vi "Linear Fit correlation.vi"(0 "Y Values":dbl[](array[numeric]) format="%.2f", 1 "X Values":dbl[](array[numeric]) format="%.2f") -> (2 "slope":dbl format="%.2f", 3 "intercept":dbl format="%.2f", 4 "r":dbl format="%.6f", 5 "error":i32)   [LabVIEW 2015]
doc: "Finds the set of linear fit coefficients slope and intercept, which describe the line that best represents the input data set. The general form of the linear fit is given by\n\n F = mX + b.\n\n where\n F is the line values that best represents the input data set.\n X is the input sequence X Values\n m is the slope\n b is the intercept."
panel:
  # "Linear Fit Coefficients"
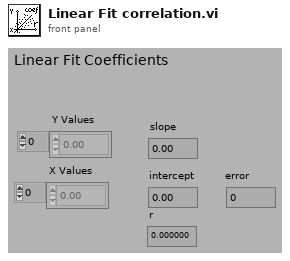
[diagram p1: front panel]
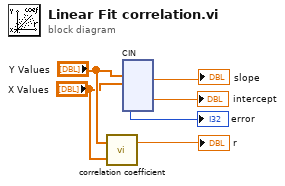
[diagram p0: block diagram]
diagram:
  n1 = call "correlation coefficient.vi"("X Values"="X Values", "Y Values"="Y Values") -> ("r"=→"r":dbl)  [unwired: 1 in]
  n2 = cin("Y Values", "X Values") -> (→"slope":dbl, →"intercept":dbl, →"error":i32)  [unwired: 5 in]
